vi "SendStartup.vi"(8 "error in (no error)":errorcluster, 10 "Sender name":string, 11 "BaseDriver in":refnum<class "BaseDriver.lvclass">) -> (0 "error out":errorcluster, 3 "BaseDriver out":refnum<class "BaseDriver.lvclass">)   [LabVIEW 2013, in "BaseDriver.lvclass"]
doc: "Sends a message from a dynamically started driver, indicating that it is alive and what responder name it will use"
uses:
  BaseDriver.lvclass
  response.ctl
  driver_status.ctl
  BaseDriver.lvclass/BaseDriver.ctl
  Responder/BaseResponder/BaseResponder.lvclass
  Responder/BaseResponder/Write Name.vi
panel:
  in  "response":T1
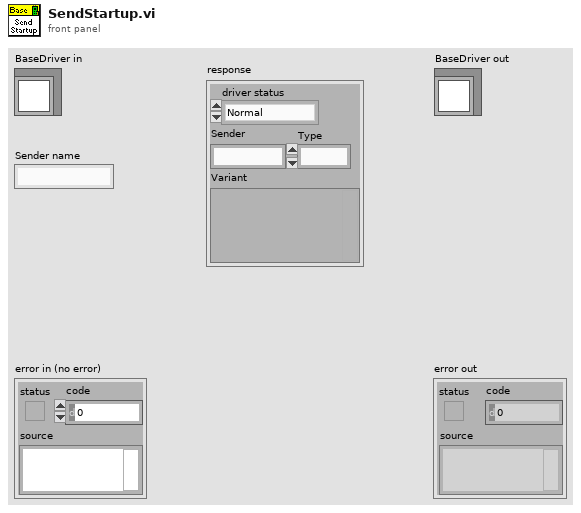
[diagram p1: front panel]
types:
  T1 = typedef "response.ctl" = cluster{"driver status":T2, "Sender":string, "Type":i32, "Variant":variant}
  T2 = typedef "driver_status.ctl" = enum16{"Normal", "Startup", "Connection lost", "Reconnected", "Timeout", "Idle", "Busy"}
  T3 = typedef "message_queue.ctl" = refnum<queue>
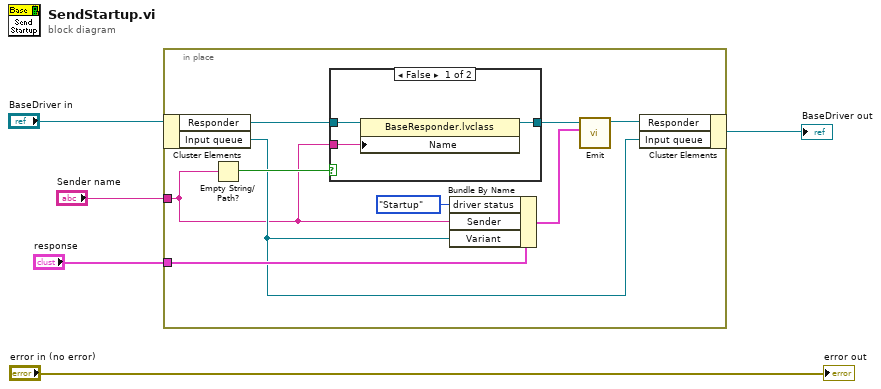
[diagram p0: block diagram]
diagram:
  n1 = in-place "In Place Element Structure" {
    in-place-border: "response" -> [w12]
    in-place-border: "Sender name" -> [w6]
    n2 = in-place-cluster #1("BaseDriver in") -> ("Responder"=w14:refnum<class "BaseResponder.lvclass">, "Input queue"=w7:T3)
    n3 = Empty String/Path?(string/path=w6) -> (empty?=w8:bool)
    n4 = case shown="False" w8 {
      tunnel: w14 -> [w17 w18]
      tunnel: [w16 w18] -> w10
      tunnel: w6 -> [w15 _]
      frame False {
        n5 = property on="Property Node" class="BaseResponder.lvclass"(reference=w17, "Name"=w15) -> (reference out=w16:refnum<class "BaseResponder.lvclass">)  [unwired: 1 in, 1 out]
      }
      frame True {
      }
    }
    n6 = Bundle By Name(cluster=w12, "driver status"=driver_status."Startup", "Sender"=w6, "Variant"=w7) -> (w9:T1)
    n7 = call-dynamic "Emit.vi"("response"=w9, "BaseResponder in"=w10) -> ("BaseResponder out"=w13:refnum<class "BaseResponder.lvclass">)  [unwired: 8 in, 1 out]
    n8 = in-place-cluster #1("Responder"=w13, "Input queue"=w7) -> (→"BaseDriver out":refnum<class "BaseDriver.lvclass">)
  }
  "error out" <- "error in (no error)"
